vi "OPC UA Server - 2 Tags.vi"() -> ()   [LabVIEW 2017]
uses:
  <vilib>/OPCUA/NI OPC UA Server.lvlib
panel:
  out "Item Node Id 2":string="ns=2;s=Process Data.TemperatureF"
  out "Item Node Id":string="ns=2;s=Process Data.TemperatureC"
  in  "Stop Button":bool
  out "Server Endpoint URL":string="opc.tcp://XPS15HPH:49580"
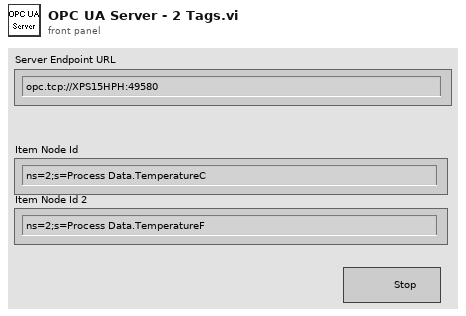
[diagram p1: front panel]
types:
  T1 = cluster{"name":string, "data type":u16, "access level":u16, "description":string}
  T2 = typedef "OPC UA Server Refnum.ctl" = refnum<k21>
  T3 = typedef "NodeId.ctl" = string
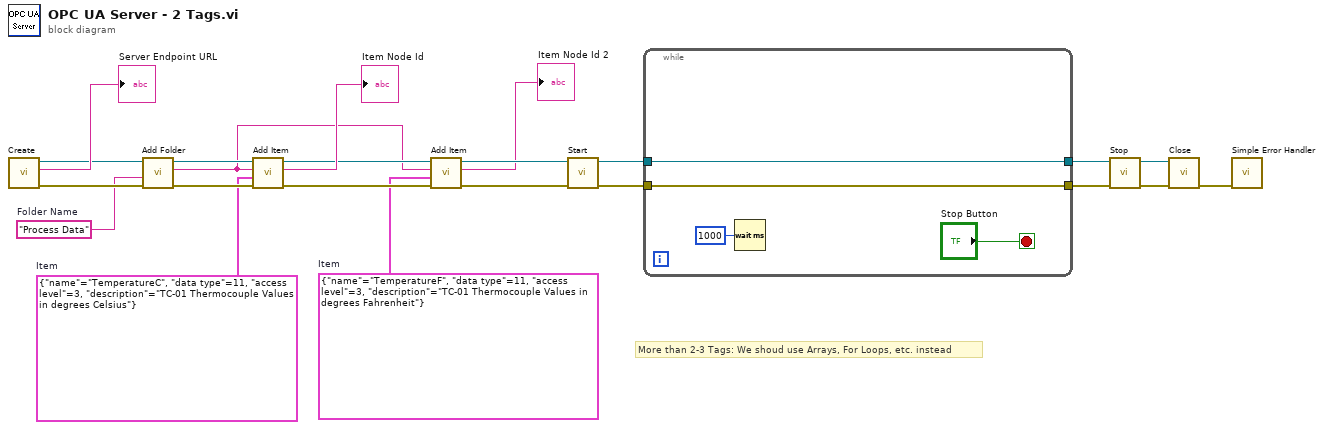
[diagram p0: block diagram]
diagram:
  w2 = T1 {"name"="TemperatureF", "data type"=11, "access level"=3, "description"="TC-01 Thermocouple Values in degrees Fahrenheit"}  # Item
  w12 = T1 {"name"="TemperatureC", "data type"=11, "access level"=3, "description"="TC-01 Thermocouple Values in degrees Celsius"}  # Item
  w16 = "Process Data"  # Folder Name
  # "More than 2-3 Tags: We shoud use Arrays, For Loops, etc. instead"
  n1 = call <vilib>:"Create.vi"() -> ("error out"=w22:errorcluster, "server endpoint URL"=→"Server Endpoint URL":string, "OPC UA server refnum out"=w15:T2)  [unwired: 9 in]
  n2 = call <vilib>:"Add Folder.vi"("error in (no error)"=w22, "folder name"=w16, "OPC UA server refnum in"=w15) -> ("error out"=w21:errorcluster, "folder node ID"=w3:T3, "OPC UA server refnum out"=w14:T2)  [unwired: 5 in]
  n3 = call <vilib>:"Add Item.vi"("error in (no error)"=w21, "item"=w12, "parent folder node ID"=w3, "OPC UA server refnum in"=w14) -> ("error out"=w5:errorcluster, "item node ID"=→"Item Node Id":T3, "OPC UA server refnum out"=w7:T2)  [unwired: 3 in, 1 out]
  n4 = call <vilib>:"Add Item.vi"("error in (no error)"=w5, "item"=w2, "parent folder node ID"=w3, "OPC UA server refnum in"=w7) -> ("error out"=w4:errorcluster, "item node ID"=→"Item Node Id 2":T3, "OPC UA server refnum out"=w6:T2)  [unwired: 3 in, 1 out]
  n5 = call <vilib>:"Start.vi"("error in (no error)"=w4, "OPC UA server refnum in"=w6) -> ("error out"=w20:errorcluster, "OPC UA server refnum out"=w13:T2)  [unwired: 7 in, 1 out]
  n6 = while {
    tunnel: w20 -> [w23]
    tunnel: w13 -> [w24]
    tunnel: [w24] -> w9
    tunnel: [w23] -> w8
    stop <- "Stop Button" stop-if-true
    n7 = Wait (ms)(milliseconds to wait=u32 1000) -> ()  [unwired: 1 out]
  }
  n8 = call <vilib>:"Stop.vi"("error in (no error)"=w8, "OPC UA server refnum in"=w9) -> ("error out"=w18:errorcluster, "OPC UA server refnum out"=w11:T2)  [unwired: 8 in]
  n9 = call <vilib>:"Close.vi"("error in (no error)"=w18, "OPC UA server refnum in"=w11) -> ("error out"=w17:errorcluster)  [unwired: 9 in]
  n10 = call <vilib>:"Simple Error Handler.vi"("error in (no error)"=w17) -> ()  [unwired: 4 in, 5 out]
